vi "status of worker1.vi"() -> ()   [LabVIEW 2020]
panel:
  out "worker1_busy/ready":bool
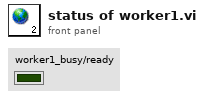
[diagram p1: front panel]
diagram:
